vi "Calculatrice 1&2.vi"() -> ()   [LabVIEW 2020]
doc: "Calculatrice 1"
panel:
  out "Intermediaire":string
  in  "entrée d'erreur (pas d'erreur)":errorcluster
  out "error out":errorcluster
  in  "Btn_Erreur ?":bool
  in  "Btn_Arrêter":bool
  out "Ind_Display":T1
  in  "Cmd_Operateur":T2
  in  "Cmd_Pad":T3
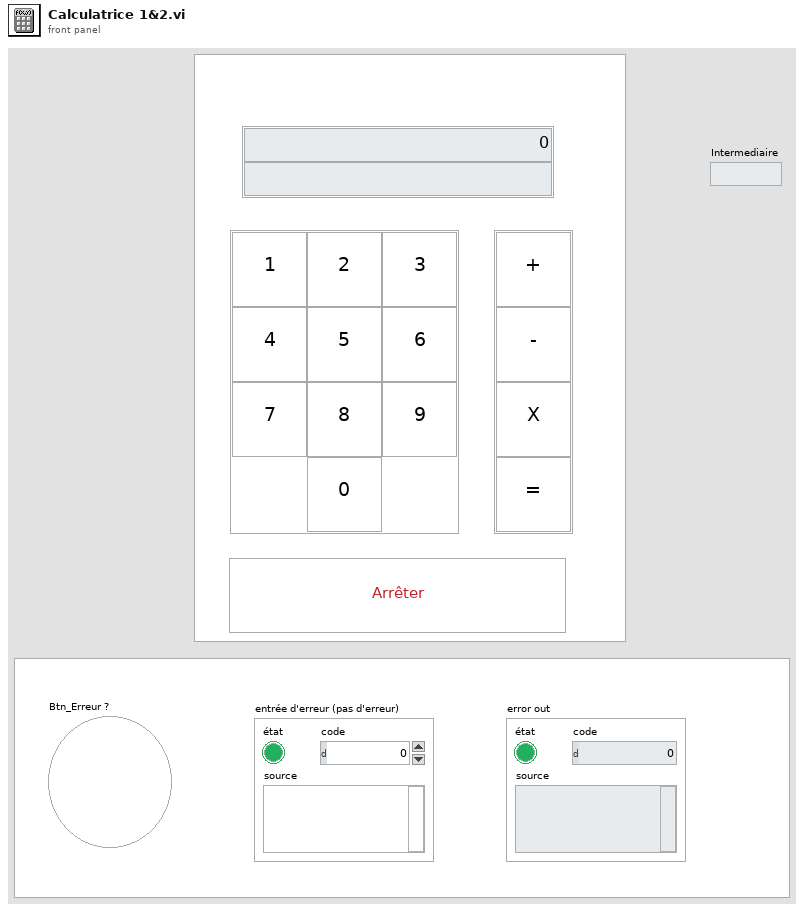
[diagram p1: front panel]
types:
  T1 = cluster{"Display_Numérique":dbl, "Display_Chaine":string}
  T2 = cluster{"Btn_+":bool, "Btn_-":bool, "Btn_X":bool, "Btn_=":bool}
  T3 = cluster{"Btn_1":bool, "Btn_2":bool, "Btn_3":bool, "Btn_4":bool, "Btn_5":bool, "Btn_6":bool, "Btn_7":bool, "Btn_8":bool, "Btn_9":bool, "Btn_10":bool}
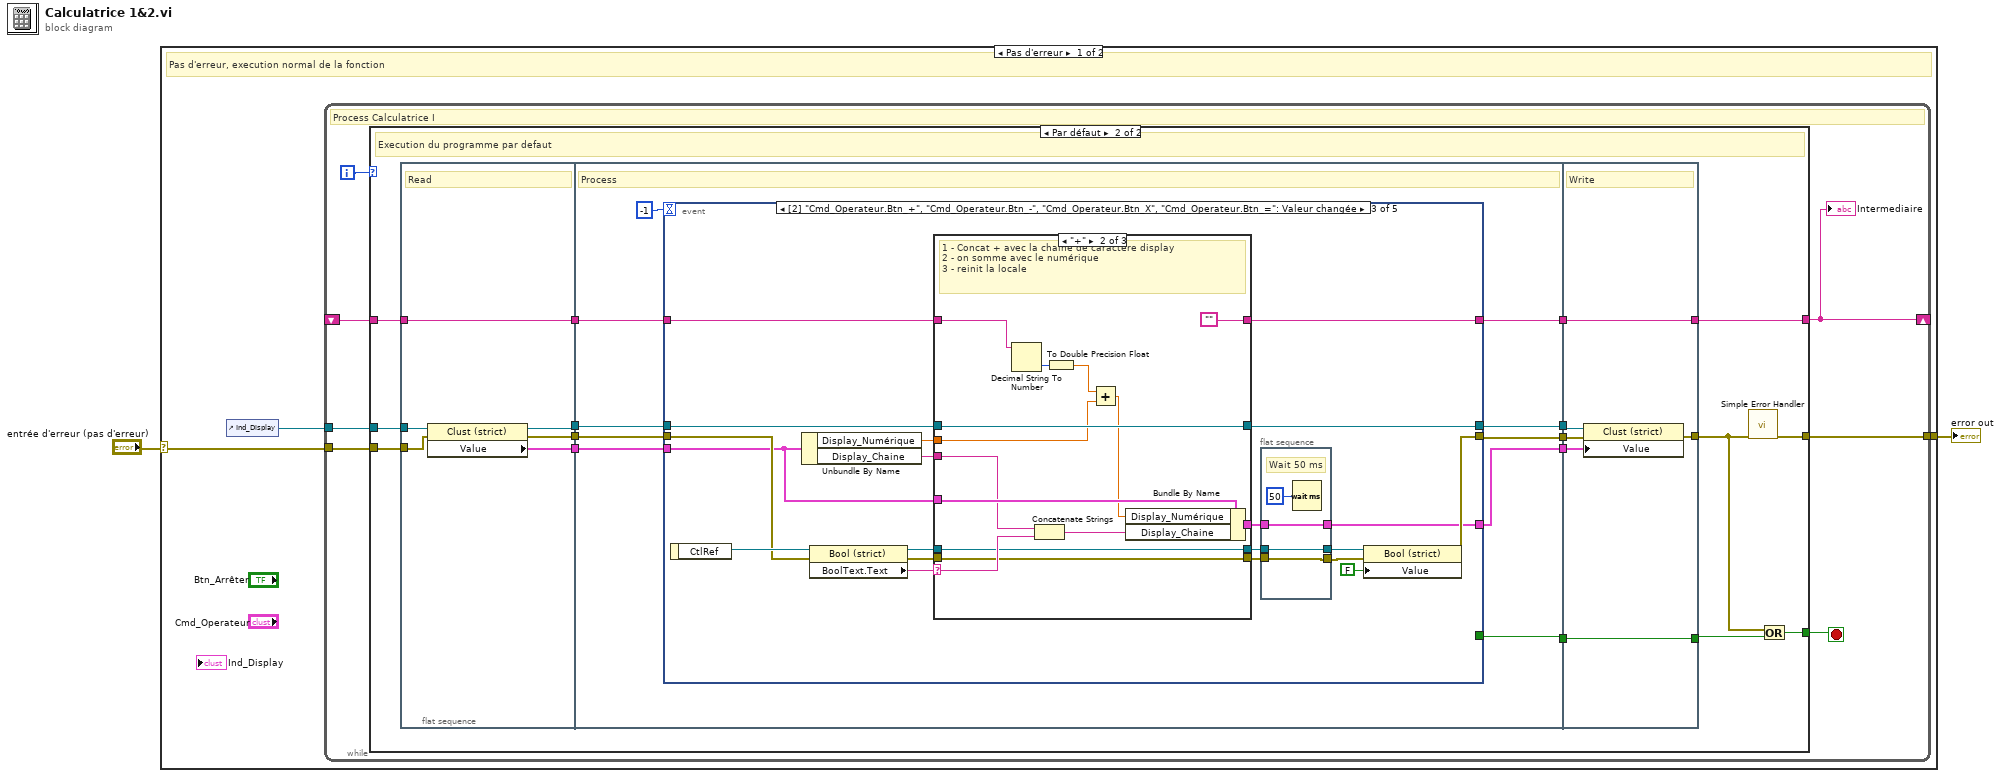
[diagram p0: block diagram]
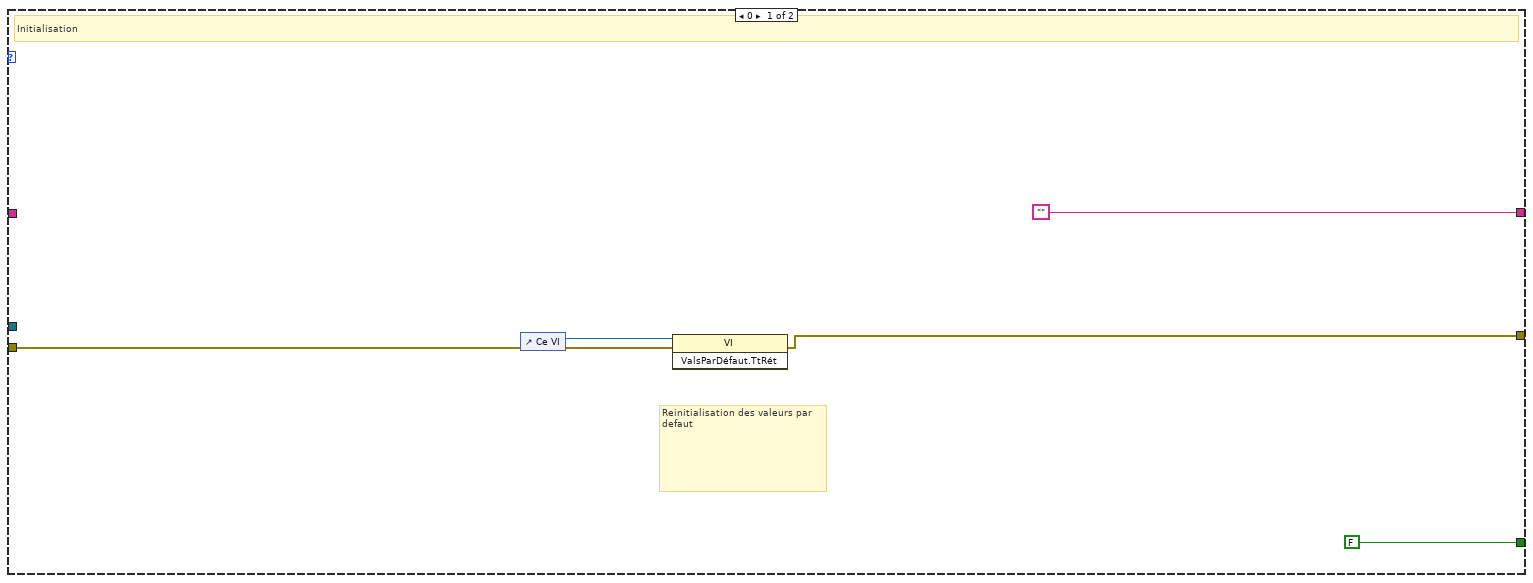
[diagram p2: hidden frame]
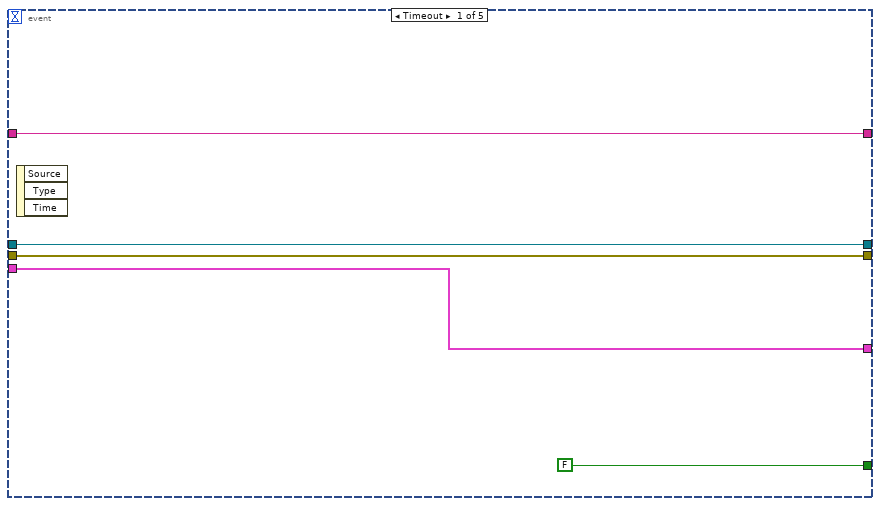
[diagram p3: hidden frame]
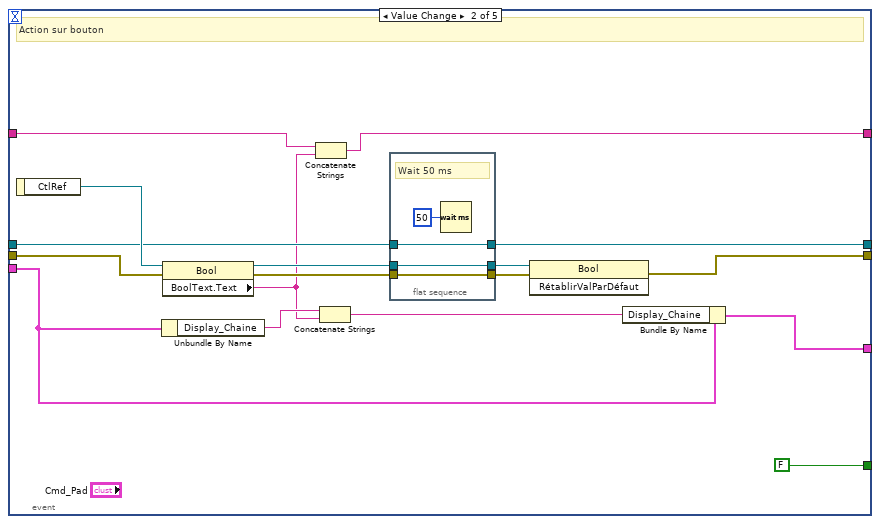
[diagram p4: hidden frame]
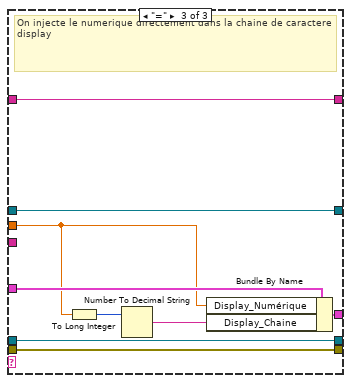
[diagram p6: hidden frame]
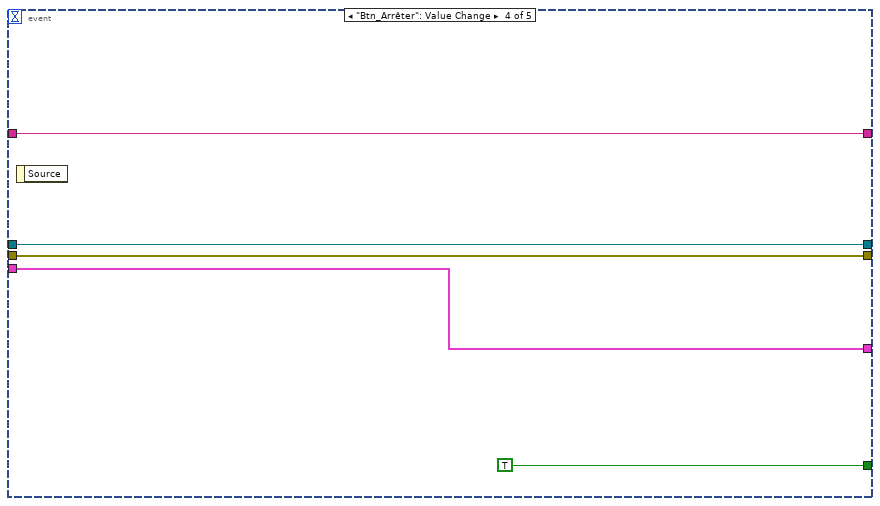
[diagram p7: hidden frame]
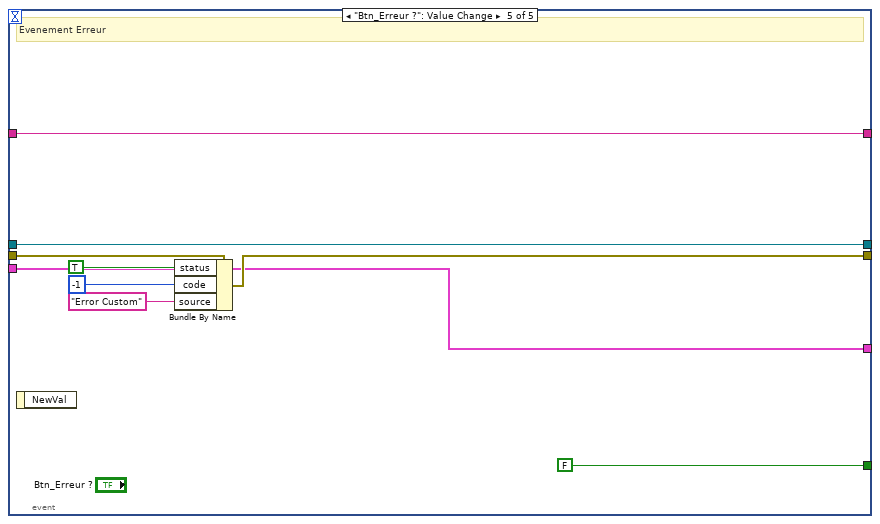
[diagram p8: hidden frame]
diagram:
  n1 = case shown="Pas d'erreur" "entrée d'erreur (pas d'erreur)" {
    selector: "entrée d'erreur (pas d'erreur)" -> [w3 w149]
    tunnel: [w4 w149] -> w2
    frame No Error {
      # "Pas d'erreur, execution normal de la fonction"
      n2 = control-ref of="Ind_Display"() -> (w5:refnum<vi>)
      n3 = while {
        tunnel: w5 -> [w12]
        tunnel: [w9] -> w4
        tunnel: w3 -> [w10]
        shift-right: [w7] -> _
        shift-left: _ -> [w6]
        i -> [w8]
        stop <- w11 stop-if-true
        # "Process Calculatrice I"
        n4 = case shown="Par défaut" w8 {
          tunnel: w12 -> [_ w27]
          tunnel: [FALSE w25] -> w11
          tunnel: w10 -> [w15 w24]
          tunnel: [w14 w22] -> w9
          tunnel: ["" w18] -> w7
          tunnel: w6 -> [_ w21]
          frame 0 {
            # "Reinitialisation des valeurs par defaut"
            # "Initialisation"
            n5 = control-ref of="Ce VI"() -> (w16:refnum<vi>)
            n6 = invoke class="VI" method="ValsParDéfaut.TtRét"(reference=w16, error in=w15) -> (error out=w14:errorcluster)  [unwired: 1 in, 2 out]
          }
          frame Default {
            # "Execution du programme par defaut"
            n7 = flat-sequence {
              tunnel: w27 -> [w40]
              tunnel: [w39] -> w34
              tunnel: [w38] -> w33
              tunnel: w24 -> [w37]
              tunnel: [w36] -> w32
              tunnel: w21 -> [w35]
              tunnel: [w35] -> w20
              tunnel: [w49] -> w31
              tunnel: w34 -> [w48]
              tunnel: [w47] -> w30
              tunnel: w33 -> [w46]
              tunnel: [w45] -> w29
              tunnel: w32 -> [w44]
              tunnel: [w43] -> w28
              tunnel: w20 -> [w42]
              tunnel: [w41] -> w19
              tunnel: [w148] -> w26
              tunnel: w31 -> [w148]
              tunnel: w30 -> [w147]
              tunnel: w29 -> [w146]
              tunnel: [w145] -> w23
              tunnel: w28 -> [w144]
              tunnel: w19 -> [w143]
              tunnel: [w143] -> w18
              frame #0 {
                # "Read"
                n8 = property class="Clust (strict)"(reference=w40, error in=w37) -> (reference out=w39:refnum<vi>, error out=w38:errorcluster, "Value"=w36:T1)
              }
              frame #1 {
                # "Process"
                n9 = event shown="[2] \"Cmd_Operateur.Btn_+\", \"Cmd_Operateur.Btn_-\", \"Cmd_Operateur.Btn_X\", \"Cmd_Operateur.Btn_=\": Valeur changée" {
                  selector: _ -> [_ _ _ _ _]
                  dyn-events: _ -> [_ _ _ _ _]
                  timeout: -1 -> [_ _ _ _ _]
                  tunnel: [FALSE FALSE _ TRUE FALSE] -> w49
                  tunnel: w48 -> [w54 w64 w92 w132 w142]
                  tunnel: [w54 w63 w91 w132 w142] -> w47
                  tunnel: w46 -> [w53 w70 w95 w131 w141]
                  tunnel: [w53 w68 w83 w131 w140] -> w45
                  tunnel: w44 -> [w52 w59 w90 w130 w135]
                  tunnel: [w52 w69 w81 w130 w135] -> w43
                  tunnel: w42 -> [w51 w61 w88 w129 w134]
                  tunnel: [w51 w60 w87 w129 w134] -> w41
                  event Timeout {
                    n10 = event-data() -> ()  [unwired: 1 in, 3 out]
                  }
                  event "Cmd_Pad.Btn_1", "Cmd_Pad.Btn_2", "Cmd_Pad.Btn_3", "Cmd_Pad.Btn_4", "Cmd_Pad.Btn_5", "Cmd_Pad.Btn_6", "Cmd_Pad.Btn_7", "Cmd_Pad.Btn_8", "Cmd_Pad.Btn_9", "Cmd_Pad.Btn_10": Value Change {
                    # "Action sur bouton"
                    n11 = event-data() -> ("CtlRef"=w71:refnum<vi>)  [unwired: 1 in]
                    n12 = Unbundle By Name(w59) -> ("Display_Chaine"=w58:string)
                    n13 = property class="Bool"(reference=w71, error in=w70) -> (reference out=w62:refnum<vi>, error out=w67:errorcluster, "BoolText.Text"=w57:string)
                    n14 = Concatenate Strings(w61, w57) -> (w60:string)
                    n15 = Concatenate Strings(w58, w57) -> (w56:string)
                    n16 = flat-sequence {
                      tunnel: w67 -> [w75]
                      tunnel: [w75] -> w66
                      tunnel: w62 -> [w74]
                      tunnel: [w74] -> w65
                      tunnel: w64 -> [w73]
                      tunnel: [w73] -> w63
                      frame #0 {
                        # "Wait 50 ms"
                        n17 = Wait (ms)(milliseconds to wait=u32 50 ("attente (ms)")) -> ()  [unwired: 1 out]
                      }
                    }
                    n18 = invoke class="Bool" method="RétablirValParDéfaut"(reference=w65, error in=w66) -> (error out=w68:errorcluster)  [unwired: 1 in, 2 out]
                    n19 = Bundle By Name(cluster=w59, "Display_Chaine"=w56) -> (w69:T1)
                  }
                  event "Cmd_Operateur.Btn_+", "Cmd_Operateur.Btn_-", "Cmd_Operateur.Btn_X", "Cmd_Operateur.Btn_=": Value Change {
                    n20 = event-data() -> ("CtlRef"=w96:refnum<vi>)  [unwired: 1 in]
                    n21 = Unbundle By Name(w90) -> ("Display_Numérique"=w86:dbl, "Display_Chaine"=w89:string)
                    n22 = property class="Bool (strict)"(reference=w96, error in=w95) -> (reference out=w85:refnum<vi>, error out=w93:errorcluster, "BoolText.Text"=w94:string)
                    n23 = case shown="\"+\"" w94 {
                      selector: w94 -> [_ w108 _]
                      tunnel: w93 -> [w101 w106 w120]
                      tunnel: w92 -> [w105 w119 w128]
                      tunnel: [w105 w119 w128] -> w91
                      tunnel: w90 -> [w104 w118 w127]
                      tunnel: w89 -> [_ w109 _]
                      tunnel: [w104 w116 w126] -> w82
                      tunnel: w88 -> [w103 w115 w125]
                      tunnel: [w103 "" w125] -> w87
                      tunnel: w86 -> [_ w114 w124]
                      tunnel: w85 -> [w102 w107 w121]
                      tunnel: [w102 w107 w121] -> w80
                      tunnel: [w101 w106 w120] -> w78
                      frame Default {
                        # "Defaut je ne fais rien"
                      }
                      frame "+" {
                        # "1 - Concat + avec la chaine de caractere display\n2 - on somme avec le numérique\n3 - reinit la locale"
                        n24 = Decimal String To Number(string=w115) -> (number=w113:i32)  [unwired: 2 in, 1 out]
                        n25 = Concatenate Strings(w109, w108) -> (w117:string)
                        n26 = To Double Precision Float(number=w113) -> (double precision float=w111:dbl)
                        n27 = Add(x=w111, y=w114) -> (x+y=w112:dbl)
                        n28 = Bundle By Name(cluster=w118, "Display_Numérique"=w112, "Display_Chaine"=w117) -> (w116:T1)
                      }
                      frame "=" {
                        # "On injecte le numerique directement dans la chaine de caractere display"
                        n29 = To Long Integer(number=w124) -> (32bit integer=w123:i32)
                        n30 = Number To Decimal String(number=w123) -> (decimal integer string=w122:string)  [unwired: 1 in]
                        n31 = Bundle By Name(cluster=w127, "Display_Numérique"=w124, "Display_Chaine"=w122) -> (w126:T1)
                      }
                    }
                    n32 = flat-sequence {
                      tunnel: w82 -> [w99]
                      tunnel: [w99] -> w81
                      tunnel: w80 -> [w98]
                      tunnel: [w98] -> w79
                      tunnel: w78 -> [w97]
                      tunnel: [w97] -> w77
                      frame #0 {
                        # "Wait 50 ms"
                        n33 = Wait (ms)(milliseconds to wait=u32 50 ("attente (ms)")) -> ()  [unwired: 1 out]
                      }
                    }
                    n34 = property class="Bool (strict)"(reference=w79, error in=w77, "Value"=FALSE ("Valeur")) -> (error out=w83:errorcluster)  [unwired: 1 out]
                  }
                  event "Btn_Arrêter": Value Change {
                    n35 = event-data() -> ()  [unwired: 1 in, 1 out]
                  }
                  event "Btn_Erreur ?": Value Change {
                    # "Evenement Erreur"
                    n36 = event-data() -> ()  [unwired: 1 in, 1 out]
                    n37 = Bundle By Name(cluster=w141, "status"=TRUE, "code"=-1, "source"="Error Custom") -> (w140:errorcluster)
                  }
                }
              }
              frame #2 {
                # "Write"
                n38 = property class="Clust (strict)"(reference=w147, error in=w146, "Value"=w144) -> (error out=w145:errorcluster)  [unwired: 1 out]
              }
            }
            n39 = call <vilib>:"Simple Error Handler.vi"("error in (no error)"=w23) -> ("error out"=w22:errorcluster)  [unwired: 4 in, 4 out]
            n40 = Or(x=w23, y=w26) -> (x .or. y?=w25:bool)
          }
        }
        "Intermediaire" <- w7
      }
    }
    frame Error {
      # "Erreur, je laisse passer le flux sans executer ma fonction"
    }
  }
  "error out" <- w2
